vi "Create from Handle.vi"(8 "error in (no error)":errorcluster, 11 "Handle":refnum<data-value>) -> (0 "error out":errorcluster, 3 "Buffer out":refnum<class "Buffer.lvclass">)   [LabVIEW 2020, in "Buffer.lvclass"]
uses:
  Buffer.lvclass
  Buffer.lvclass/Buffer.ctl
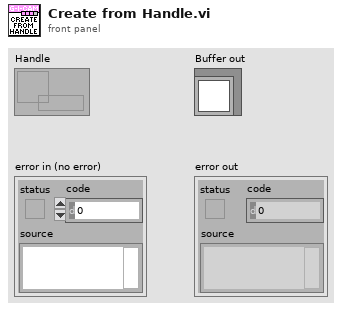
[diagram p1: front panel]
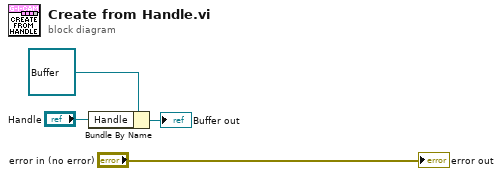
[diagram p0: block diagram]
diagram:
  n1 = Bundle By Name(cluster=refnum<class "Buffer.lvclass"> refnum ("Buffer in"), "Handle"="Handle") -> (→"Buffer out":refnum<class "Buffer.lvclass">)
  "error out" <- "error in (no error)"
